vi "Fetch.vi"(8 "error in":errorcluster, 10 "Display":string(combo), 11 "VISA resource name in":refnum<visa-resource-name>) -> (0 "error out":errorcluster, 2 "Value":dbl, 3 "VISA resource name out":refnum<visa-resource-name>)   [LabVIEW 2021, in "Keysight U1282A.lvlib"]
doc: "El comando FETC? regresa el valor de la pantalla principal, secundaria o temperatura."
uses:
  Keysight U1282A.lvlib
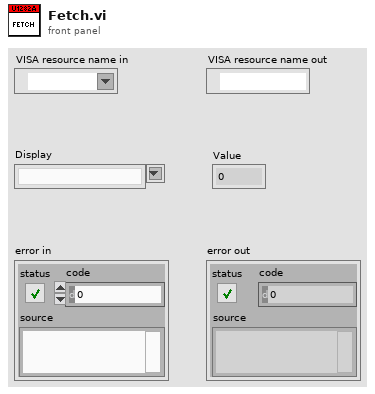
[diagram p1: front panel]
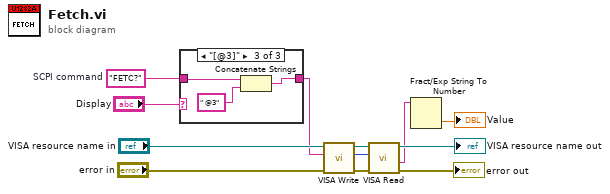
[diagram p0: block diagram]
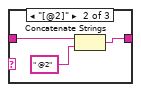
[diagram p3: hidden frame]
diagram:
  w4 = "FETC?"  # SCPI command
  n1 = case shown="\"[@3]\"" "Display" {
    tunnel: w4 -> [w13 w15 w18]
    tunnel: [w13 w14 w17] -> w3
    frame Default {
    }
    frame "[@2]" {
      n2 = Concatenate Strings(w15, " @2") -> (w14:string)
    }
    frame "[@3]" {
      n3 = Concatenate Strings(w18, " @3") -> (w17:string)
    }
  }
  n4 = call "VISA Write.vi"("error in"="error in", "SCPI command"=w3, "VISA resource in"="VISA resource name in") -> ("error out"=w12:errorcluster, "Bytes at Port out"=w6:u32, "VISA resource out"=w7:refnum<visa-resource-name>)  [unwired: 6 in]
  n5 = call "VISA Read.vi"("error in"=w12, "Bytes at Port in"=w6, "VISA resource in"=w7) -> ("error out"=→"error out":errorcluster, "Reading"=w1:string, "VISA resource out"=→"VISA resource name out":refnum<visa-resource-name>)  [unwired: 5 in, 1 out]
  n6 = Fract/Exp String To Number(string=w1) -> (number=→"Value":dbl)  [unwired: 3 in, 1 out]
